vi "Vision Processing.vi"(8 "error in (no error)":errorcluster, 11 "Image Size":T1=enum."320x240") -> ()   [LabVIEW 2016]
uses:
  Vision Support Code/Camera Types.ctl
  <vilib>/Rock Robotics/WPI/Camera/WPI_CameraImageSize.ctl
  <vilib>/Rock Robotics/WPI/Camera/WPI_CameraWhite Balance Values.ctl
  <vilib>/Rock Robotics/WPI/Camera/WPI_CameraFrameRate.ctl
  <vilib>/Rock Robotics/WPI/Camera/WPI_CameraExposure Values.ctl
  Robot Global Data.vi
  <vilib>/Rock Robotics/Network Tables/NT Write Number.vi
  <vilib>/vision/NI_Vision_Development_Module.lvlib
panel:
  in  "Image Size 2":T1=enum."320x240"
  out "loop ms":u32=100
  out "Calibration error":errorcluster={"status"=TRUE, "code"=-1074396113, "source"=""}
  in  "Display Original":bool=TRUE
  in  "Display Mask":bool=TRUE
  in  "Line Border":cluster{"Top":dbl, "Bottom":dbl}={"Top"=6.0, "Bottom"=1.0}
  in  "Use Calibration":bool=TRUE
  out "Instructions:":string="Use Source to load image files from a directory, or use a USB or IP camera connected to your laptop. Use Camera Settings 1 and 2 to achieve a dark image with bright and colorful stripes.\nLED Color can encoded as HSL or related color modes. Calibrate to the same color as the strips being reflected to the camera.\nClick and draw a line in Original Image to auto-calibrate the LED Color. You may want to widen and tweak Sat and Val by hand.\nThe Annotate button affects drawing a rectangle around the stripes and labeling it with a distance in ft. Distance relies on knowing the Camera Type and lens calibration (it looks up the lens view angle).\n\nAdjust Score Cutoff to make the code more or less picky. If the color is not very unique, you may need to increase the number of particles considered. The diagram uses a Size Limit to ignore colored things that are too small. You may need to adjust it if you are targetting from far away.\n\nResults give you the distance to the target, the center and box in a normalized (-1 to 1) and pixel coordinates.\n\nBe sure to read about setting camera exposure and brightness to help simplify your image and acquire color saturated images.\n\nThere are lots of comments on the diagram to explain the code."
  in  "Color Mode":u16(ring)=3 items=["RGB", "HSL", "HSV", "HSI"]
  in  "Particles":dbl=5.0
  in  "Score Cutoff %":dbl=70.0
  in  "Camera Type":T2=enum."MS HD3000 square"
  out "Results":T3={"Distance (ft)"=inf, "Score"=32.16524216524216, "Normalized"={"Center"={0.9161960132890365, 0.41043743078626804}, "Rectangle"={"Numeric"=0.6062500000000002, "Numeric 2"=0.525, "Numeric 3"=0.9625000000000001, "Numeric 5"=0.275}}, "Pixels"={"Center"={306.5913621262458, 70.74750830564784}, "Rectangle"={"Numeric"=257.0, "Numeric 2"=57.0, "Numeric 3"=314.0, "Numeric 5"=87.0}}} {"Score" format="%#_3g"; "Pixels"."Rectangle"."Numeric 5" format="%#_3g"; "Pixels"."Rectangle"."Numeric 3" format="%#_3g"; "Pixels"."Rectangle"."Numeric 2" format="%#_3g"; "Pixels"."Rectangle"."Numeric" format="%#_3g"; "Normalized"."Rectangle"."Numeric 5" format="%#_2g"; "Normalized"."Rectangle"."Numeric 3" format="%#_2g"; "Normalized"."Rectangle"."Numeric 2" format="%#_2g"; "Normalized"."Rectangle"."Numeric" format="%#_2g"; "Normalized"."Center"."?" format="%#_3g"; "Normalized"."Center"."?" format="%#_3g"; "Distance (ft)" format="%#_3g"}
  out "Qualified Particles":i32=2
  in  "LED Color":T4={"Hue"={46.852959751357716, 98.19702858546475}, "Sat"={45.53571428571429, 255.0}, "Val"={40.53571428571429, 255.0}} {"Hue" scale=0.0..255.0 scale format="%#_3g"}
  out "Mask":T5(plugin-control)
  out "Original Image":T5(plugin-control)
  # "Legend:\n    Rectangle\n       Green - Good target, distance ft\n       Red - Bad target\n    Orange Text - Score in %"
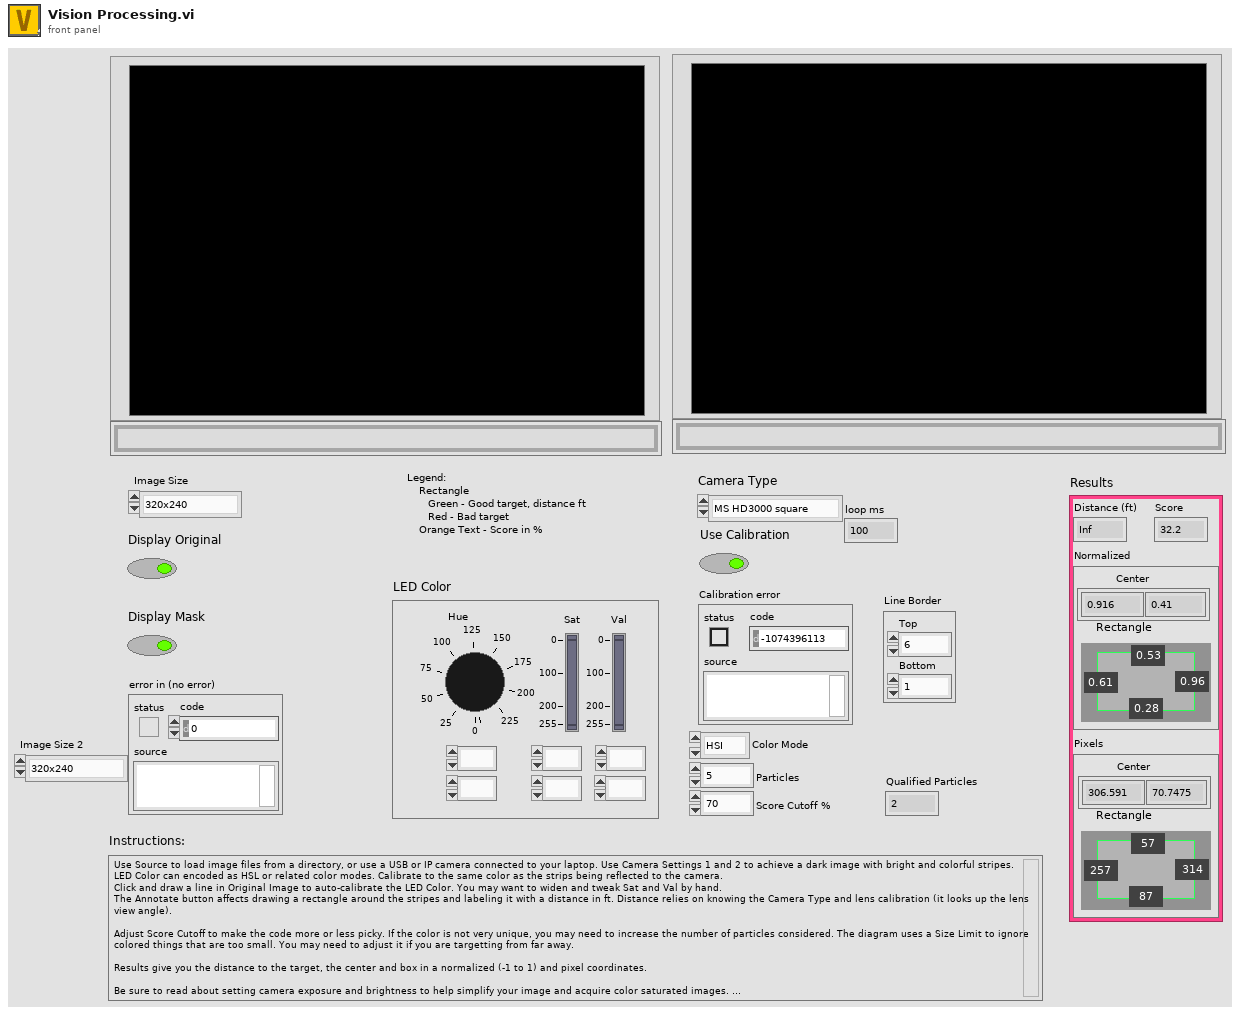
[diagram p1: front panel]
types:
  T1 = typedef "WPI_CameraImageSize.ctl" = enum16{"640x480", "320x240", "160x120", "Custom"}
  T2 = typedef "Camera Types.ctl" = enum16{"206", "1011", "1013", "MS HD3000 square", "MS HD3000 640x480"}
  T3 = cluster{"Distance (ft)":dbl, "Score":dbl, "Normalized":cluster{"Center":cluster{dbl, dbl}, "Rectangle":cluster{"Numeric":dbl, "Numeric 2":dbl, "Numeric 3":dbl, "Numeric 5":dbl}}, "Pixels":cluster{"Center":cluster{dbl, dbl}, "Rectangle":cluster{"Numeric":dbl, "Numeric 2":dbl, "Numeric 3":dbl, "Numeric 5":dbl}}}
  T4 = cluster{"Hue":cluster{dbl, dbl}, "Sat":cluster{dbl, dbl}, "Val":cluster{dbl, dbl}}
  T5 = typedef "IMAQ Image.ctl" = refnum<image>
  T6 = typedef "WPI_CameraFrameRate.ctl" = u32
  T7 = typedef "WPI_CameraExposure Values.ctl" = enum16{"Auto", "Flicker-free 50 Hz", "Flicker-free 60 Hz", "Hold current", "Custom"}
  T8 = typedef "WPI_CameraWhite Balance Values.ctl" = enum16{"Auto", "Fixed indoor", "Fixed outdoor 1", "Fixed outdoor 2", "Fixed fluorescent 1", "Fixed fluorescent 2", "Hold current", "Custom"}
  T9 = typedef "Image Type" = u32
  T10 = typedef "Particle Parameters" = i32
  T11 = typedef "WPI_CameraDevRef.ctl" = cluster{"Camera Address":string, "CameraStatus":errorcluster}
  T12 = cluster{"Left":dbl, "Top":dbl, "Right":dbl, "Bottom":dbl}
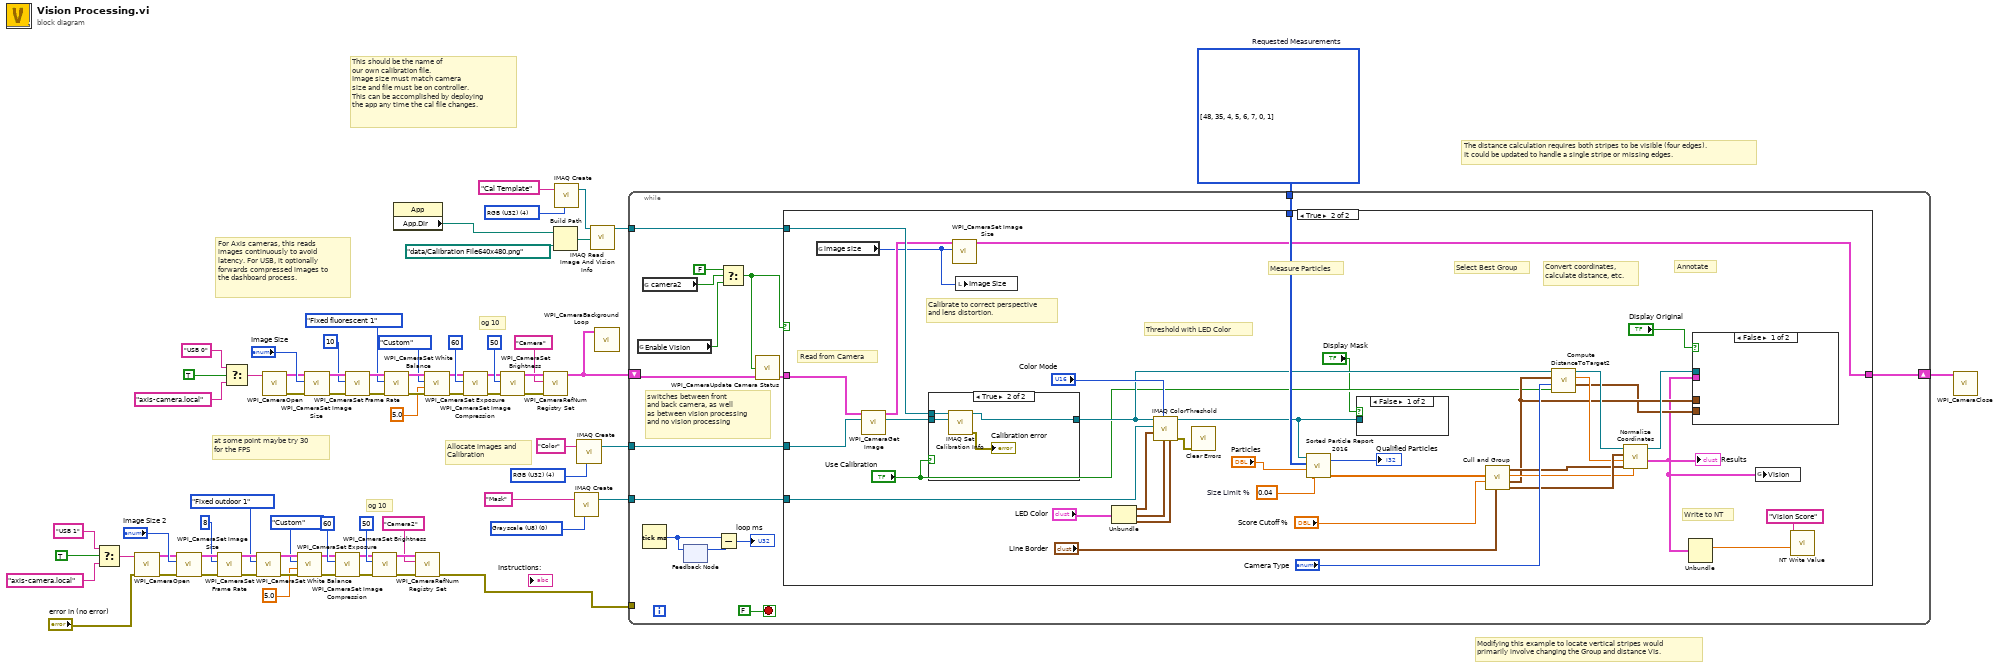
[diagram p0: block diagram]
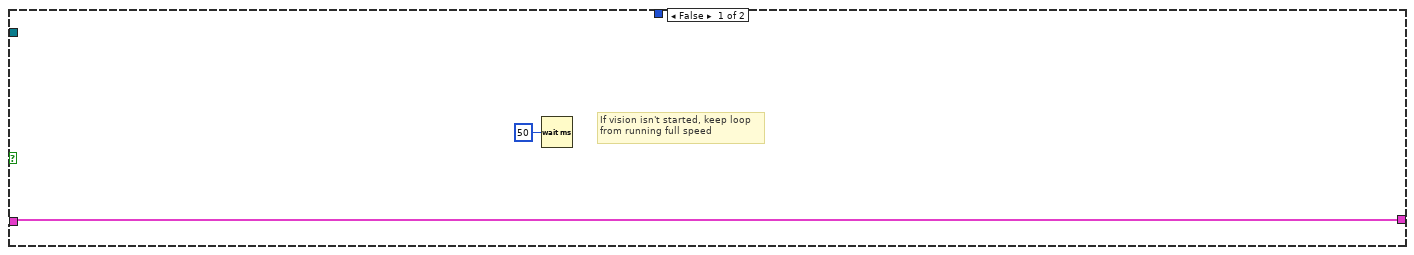
[diagram p2: hidden frame]
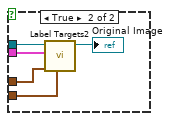
[diagram p3: hidden frame]
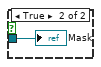
[diagram p4: hidden frame]
diagram:
  w63 = T9 4 items=["Grayscale (U8)", "Grayscale (I16)", "Grayscale (SGL)", "Complex (CSG)", "RGB (U32)", "HSL (U32)", "RGB (U64)", "Grayscale (U16)"] ("Image Type")
  w65 = T10[] [48, 35, 4, 5, 6, 7, 0, 1] items=["Center of Mass X", "Center of Mass Y", "First Pixel X", "First Pixel Y", "Bounding Rect Left", "Bounding Rect Top", "Bounding Rect Right", "Bounding Rect Bottom", "Max Feret Diameter Start X", "Max Feret Diameter Start Y", "Max Feret Diameter End X", "Max Feret Diameter End Y", "Max Horiz. Segment Length Left", "Max Horiz. Segment Length Right", "Max Horiz. Segment Length Row", "-", "Bounding Rect Width", "Bounding Rect Height", "Bounding Rect Diagonal", "Perimeter", "Convex Hull Perimeter", "Holes' Perimeter", "Max Feret Diameter", "Equivalent Ellipse Major Axis", "Equivalent Ellipse Minor Axis", "Equivalent Ellipse Minor Axis (Feret)", "Equivalent Rect Long Side", "Equivalent Rect Short Side", "Equivalent Rect Diagonal", "Equivalent Rect Short Side (Feret)", "Average Horiz. Segment Length", "Average Vert. Segment Length", "Hydraulic Radius", "Waddel Disk Diameter", "-", "Area", "Holes' Area", "Particle & Holes' Area", "Convex Hull Area", "Image Area", "-", "Number of Holes", "Number of Horiz. Segments", "Number of Vert. Segments", "-", "Orientation", "Max Feret Diameter Orientation", "-", "% Area/Image Area", "% Area/(Particle & Holes' Area)", "Ratio of Equivalent Ellipse Axes", "Ratio of Equivalent Rect Sides", "-", "Elongation Factor", "Compactness Factor", "Heywood Circularity Factor", "Type Factor", "-", "Sum X", "Sum Y", "Sum XX", "Sum XY", "Sum YY", "Sum XXX", "Sum XXY", "Sum XYY", "Sum YYY", "-", "Moment of Inertia XX", "Moment of Inertia XY", "Moment of Inertia YY", "Moment of Inertia XXX", "Moment of Inertia XXY", "Moment of Inertia XYY", "Moment of Inertia YYY", "Norm. Moment of Inertia XX", "Norm. Moment of Inertia XY", "Norm. Moment of Inertia YY", "Norm. Moment of Inertia XXX", "Norm. Moment of Inertia XXY", "Norm. Moment of Inertia XYY", "Norm. Moment of Inertia YYY", "Hu Moment 1", "Hu Moment 2", "Hu Moment 3", "Hu Moment 4", "Hu Moment 5", "Hu Moment 6", "Hu Moment 7"]  # Requested Measurements
  w68 = T9 0 items=["Grayscale (U8)", "Grayscale (I16)", "Grayscale (SGL)", "Complex (CSG)", "RGB (U32)", "HSL (U32)", "RGB (U64)", "Grayscale (U16)"] ("Image Type")
  w69 = T9 4 items=["Grayscale (U8)", "Grayscale (I16)", "Grayscale (SGL)", "Complex (CSG)", "RGB (U32)", "HSL (U32)", "RGB (U64)", "Grayscale (U16)"] ("Image Type")
  # "og 10"
  # "og 10"
  # "at some point maybe try 30 \nfor the FPS"
  # "This should be the name of \nour own calibration file.\nImage size must match camera\nsize and file must be on controller.\nThis can be accomplished by deploying\nthe app any time the cal file changes."
  # "For Axis cameras, this reads\nimages continuously to avoid\nlatency. For USB, it optionally\nforwards compressed images to\nthe dashboard process."
  # "Modifying this example to locate vertical stripes would\nprimarily involve changing the Group and distance VIs."
  # "The distance calculation requires both stripes to be visible (four edges).\nIt could be updated to handle a single stripe or missing edges."
  # "Allocate images and\nCalibration"
  n1 = Select(t="USB 1" ("format string"), s=TRUE ("dot notation? (F)"), f="axis-camera.local" ("format string")) -> (s? t:f=w4:string)
  n2 = call <vilib>:"WPI_CameraOpen.vi"("error in (no error)"="error in (no error)", "Camera Address"=w4) -> ("error out"=w16:errorcluster, "CameraDevRef"=w17:T11)  [unwired: 8 out]
  n3 = call <vilib>:"WPI_CameraSet Image Size.vi"("error in (no error)"=w16, "Image Size"="Image Size 2", "CameraDevRef"=w17) -> ("error out"=w15:errorcluster, "CameraDevRef Out"=w18:T11)  [unwired: 1 in, 6 out]
  n4 = call <vilib>:"WPI_CameraSet Frame Rate.vi"("error in (no error)"=w15, "Frame Rate (fps)"=T6 8, "CameraDevRef"=w18) -> ("error out"=w14:errorcluster, "CameraDevRef Out"=w20:T11)  [unwired: 7 out]
  n5 = Select(t="USB 0" ("format string"), s=TRUE ("dot notation? (F)"), f="axis-camera.local" ("format string")) -> (s? t:f=w33:string)
  n6 = call <vilib>:"WPI_CameraSet White Balance.vi"("error in (no error)"=w14, "White Balance"=WPI_CameraWhite_Balance_Values."Fixed outdoor 1", "CameraDevRef"=w20) -> ("error out"=w13:errorcluster, "CameraDevRef Out"=w19:T11)  [unwired: 1 in, 6 out]
  n7 = call <vilib>:"WPI_CameraOpen.vi"("Camera Address"=w33) -> ("error out"=w45:errorcluster, "CameraDevRef"=w46:T11)  [unwired: 1 in, 8 out]
  n8 = call <vilib>:"WPI_CameraSet Exposure.vi"("error in (no error)"=w13, "Exposure (%)"=5.0, "Exposure"=WPI_CameraExposure_Values."Custom", "CameraDevRef"=w19) -> ("error out"=w12:errorcluster, "CameraDevRef Out"=w22:T11)  [unwired: 6 out]
  n9 = call <vilib>:"WPI_CameraSet Image Size.vi"("error in (no error)"=w45, "Image Size"="Image Size", "CameraDevRef"=w46) -> ("error out"=w44:errorcluster, "CameraDevRef Out"=w47:T11)  [unwired: 1 in, 6 out]
  n10 = call <vilib>:"WPI_CameraSet Image Compression.vi"("error in (no error)"=w12, "Compression"=60, "CameraDevRef"=w22) -> ("error out"=w11:errorcluster, "CameraDevRef Out"=w21:T11)  [unwired: 7 out]
  n11 = call <vilib>:"WPI_CameraSet Frame Rate.vi"("error in (no error)"=w44, "Frame Rate (fps)"=T6 10, "CameraDevRef"=w47) -> ("error out"=w43:errorcluster, "CameraDevRef Out"=w49:T11)  [unwired: 7 out]
  n12 = call <vilib>:"WPI_CameraSet Brightness.vi"("error in (no error)"=w11, "Brightness"=50, "CameraDevRef"=w21) -> ("error out"=w10:errorcluster, "CameraDevRef Out"=w28:T11)  [unwired: 7 out]
  n13 = call <vilib>:"WPI_CameraSet White Balance.vi"("error in (no error)"=w43, "White Balance"=WPI_CameraWhite_Balance_Values."Fixed fluorescent 1", "CameraDevRef"=w49) -> ("error out"=w42:errorcluster, "CameraDevRef Out"=w48:T11)  [unwired: 1 in, 6 out]
  n14 = property class="App"() -> ("App.Dir"=w29:path)  [unwired: 2 in, 2 out]
  n15 = call <vilib>:"WPI_CameraRefNum Registry Set.vi"("error in (no error)"=w10, "refnum name"="Camera2", "CameraDevRef"=w28) -> ("error out"=w2:errorcluster)  [unwired: 1 in, 7 out]
  n16 = call <vilib>:"WPI_CameraSet Exposure.vi"("error in (no error)"=w42, "Exposure (%)"=5.0, "Exposure"=WPI_CameraExposure_Values."Custom", "CameraDevRef"=w48) -> ("error out"=w41:errorcluster, "CameraDevRef Out"=w51:T11)  [unwired: 6 out]
  n17 = call <vilib>:"WPI_CameraSet Image Compression.vi"("error in (no error)"=w41, "Compression"=60, "CameraDevRef"=w51) -> ("error out"=w40:errorcluster, "CameraDevRef Out"=w50:T11)  [unwired: 7 out]
  n18 = call <vilib>:"WPI_CameraSet Brightness.vi"("error in (no error)"=w40, "Brightness"=50, "CameraDevRef"=w50) -> ("error out"=w39:errorcluster, "CameraDevRef Out"=w57:T11)  [unwired: 7 out]
  n19 = call <vilib>:"WPI_CameraRefNum Registry Set.vi"("error in (no error)"=w39, "refnum name"="Camera", "CameraDevRef"=w57) -> ("CameraDevRef"=w32:T11)  [unwired: 1 in, 7 out]
  n20 = Build Path(base path=w29, name or relative path=path "data/Calibration File640x480.png" ("Folder Location")) -> (appended path=w59:path)
  n21 = call "IMAQ Create"("Image Name"="Cal Template", "Image Type"=w63) -> ("New Image"=w61:T5)  [unwired: 2 in, 2 out]
  n22 = call "IMAQ Create"("Image Name"="Mask", "Image Type"=w68) -> ("New Image"=w66:T5)  [unwired: 2 in, 2 out]
  n23 = call "IMAQ Create"("Image Name"="Color", "Image Type"=w69) -> ("New Image"=w64:T5)  [unwired: 2 in, 2 out]
  n24 = call "IMAQ Read Image And Vision Info"("File Path"=w59, "Image"=w61) -> ("Image Out"=w60:T5)  [unwired: 7 in, 2 out]
  n25 = call <vilib>:"WPI_CameraBackground Loop.vi"("CameraDevRef"=w32) -> ()  [unwired: 11 in]
  n26 = while {
    tunnel: w64 -> [w81]
    tunnel: w66 -> [w84]
    tunnel: w65 -> [w83]
    tunnel: w60 -> [w82]
    shift-right: [w80] -> w31
    shift-left: w32 -> [w79]
    tunnel: w2 -> [_]
    stop <- FALSE stop-if-true
    # "switches between front\nand back camera, as well \nas between vision processing \nand no vision processing"
    n27 = global read "Robot Global Data.vi" "Enable Vision"() -> (w72:bool)
    n28 = global read "Robot Global Data.vi" "camera2"() -> (w73:bool)
    n29 = Tick Count (ms)() -> (millisecond timer value=w76:u32)
    n30 = feedback-in #1(w76) -> ()
    n31 = feedback #1() -> (w77:u32)  [unwired: 1 in]
    n32 = Subtract(x=w76, y=w77) -> (x-y=→"loop ms":u32)
    n33 = Select(t=FALSE, s=w73, f=w72) -> (s? t:f=w71:bool)
    n34 = call <vilib>:"WPI_CameraUpdate Camera Status.vi"("CameraDevRef In"=w79, "Enable Vision"=w71) -> ("CameraDevRef Out"=w78:T11)  [unwired: 3 in]
    n35 = case shown="True" w71 {
      tunnel: w84 -> [_ w125]
      tunnel: w83 -> [_ w121]
      tunnel: w82 -> [_ w101]
      tunnel: w78 -> [w87 w98]
      tunnel: w81 -> [_ w97]
      tunnel: [w87 w92] -> w80
      frame False {
        # "If vision isn't started, keep loop\nfrom running full speed"
        n36 = Wait (ms)(milliseconds to wait=u32 50) -> ()  [unwired: 1 out]
      }
      frame True {
        w119 = 0.04  # Size Limit %
        # "Write to NT"
        # "Read from Camera"
        # "Calibrate to correct perspective\nand lens distortion."
        # "Measure Particles"
        # "Convert coordinates,\ncalculate distance, etc."
        # "Annotate"
        # "Select Best Group"
        # "Threshold with LED Color"
        n37 = global read "Robot Global Data.vi" "image size"() -> (w91:T1)
        n38 = call <vilib>:"WPI_CameraGet Image.vi"("Image"=w97, "CameraDevRef"=w98) -> ("Image Out"=w96:T5, "CameraDevRef Out"=w93:T11)  [unwired: 7 in, 1 out]
        n39 = case shown="True" "Use Calibration" {
          tunnel: [w132 w136] -> w102
          tunnel: w96 -> [w132 w135]
          tunnel: w101 -> [_ w134]
          frame False {
          }
          frame True {
            n40 = call "IMAQ Set Calibration Info"("Image Dst"=w135, "Image Src"=w134) -> ("error out"=→"Calibration error":errorcluster, "Calibrated Image"=w136:T5)  [unwired: 8 in]
          }
        }
        n41 = call <vilib>:"WPI_CameraSet Image Size.vi"("Image Size"=w91, "CameraDevRef"=w93) -> ("CameraDevRef Out"=w92:T11)  [unwired: 2 in, 7 out]
        n42 = local write "Image Size"(w91) -> ()
        n43 = Unbundle("LED Color") -> ("Hue"=w124:cluster{dbl, dbl}, "Sat"=w123:cluster{dbl, dbl}, "Val"=w122:cluster{dbl, dbl})
        n44 = call "IMAQ ColorThreshold"("Blue or Luma or Val or Inten Range"=w122, "Green or Sat Range"=w123, "Color Mode"="Color Mode", "Red or Hue Range"=w124, "Image Dst"=w125, "Image Src"=w102) -> ("error out"=w118:errorcluster, "Image Dst Out"=w114:T5)  [unwired: 4 in]
        n45 = call <vilib>:"Clear Errors.vi"("error in (no error)"=w118) -> ()  [unwired: 5 in, 2 out]
        n46 = call "Sorted Particle Report 2016.vi"("Min Area Size %"=w119, "Particle Count Limit"="Particles", "Pixel Measurements"=w121, "Image in"=w114) -> ("Sorted Data"=w116:dbl[][], "Particles"=→"Qualified Particles":i32)
        n47 = case shown="False" "Display Mask" {
          tunnel: w114 -> [_ w131]
          frame False {
          }
          frame True {
            "Mask" <- w131
          }
        }
        n48 = call "Cull and Group.vi"("Line Border"="Line Border", "Score Cutoff"="Score Cutoff %", "Sorted Data"=w116) -> ("Rect"=w112:T12, "Line"=w104:T12, "Score"=w107:dbl, "Center"=w108:cluster{"X":dbl, "Y":dbl})  [unwired: 5 in]
        n49 = call "Compute DistanceToTarget2.vi"("Calibrated"="Use Calibration", "Camera Type"="Camera Type", "Line"=w104, "Image Src"=w102) -> ("Edges"=w103:cluster{"X":sgl, "Y":sgl}[], "Distance (ft)"=w111:dbl, "Image Dst Out"=w110:T5)  [unwired: 5 in]
        n50 = call "Normalize Coordinates.vi"("Score"=w107, "Center"=w108, "Distance"=w111, "Bounding box"=w112, "Image in"=w110) -> ("Results"=w88:T3, "Image out"=w109:T5)  [unwired: 5 in]
        "Results" <- w88
        n51 = Unbundle(w88) -> ("Score"=w90:dbl)  [unwired: 3 out]
        n52 = case shown="False" "Display Original" {
          tunnel: w109 -> [_ w129]
          tunnel: w88 -> [_ w128]
          tunnel: w104 -> [_ w127]
          tunnel: w103 -> [_ w126]
          frame False {
          }
          frame True {
            n53 = call "Label Targets2.vi"("Edges"=w126, "Line"=w127, "Results"=w128, "Image in"=w129) -> ("Image out"=→"Original Image":T5)  [unwired: 7 in]
          }
        }
        n54 = global write "Robot Global Data.vi" "Vision"(w88) -> ()
        n55 = call-poly <vilib>:"NT Write Value.vi"("Numeric"=w90, "Name"="Vision Score") -> ()  [unwired: 9 in, 1 out]
      }
    }
  }
  n56 = call <vilib>:"WPI_CameraClose.vi"("CameraDevRef"=w31) -> ()  [unwired: 1 in, 10 out]
